vi "Base_eleve.vi"() -> ()   [LabVIEW 2018]
uses:
  <vilib>/Instr/_visa.llb/VISA Configure Serial Port (Instr).vi
panel:
  out "Temperature (Kelvin)":dbl
  out "Temperature (Fahrenheit)":dbl
  in  "Chemin":path
  in  "Extension du fichier":string(combo)
  in  "Nom du fichier":string
  in  "OK Button":bool
  in  "PAUSE":bool
  out "Array 3":dbl[](array[numeric])
  out "Array 2":dbl[](array[numeric])
  out "Array":dbl[](array[numeric])
  out "Humidity":dbl[](graph)
  out "Pressure":dbl[](graph)
  out "Temperature":dbl[](graph)
  out "Humidity":dbl
  out "Pressure":dbl
  out "Temperature (Celsuis)":dbl
  out "Chaîne":string
  in  "stop":bool
  in  "Nom de ressource VISA":refnum<visa-resource-name>
  # "1. Brancher la carte Arduino sur un port USB\n2. Choisir le port COM de la carte dans la liste déroulante \"Nom de ressource VISA\"\n3. Lancer le programme"
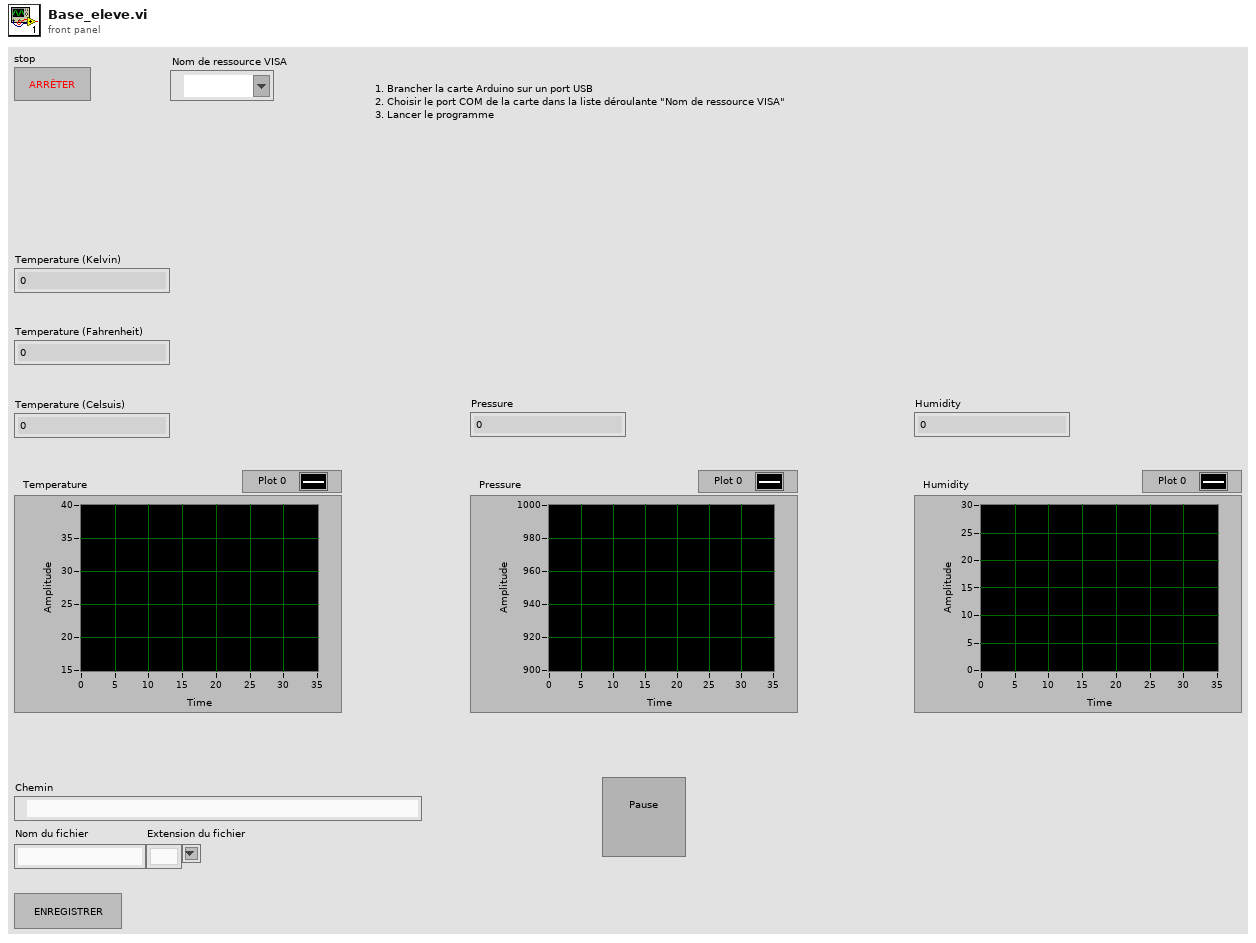
[diagram p1: front panel]
types:
  T1 = enum16{"open", "replace", "create", "open or create", "replace or create", "replace or create with confirmation"}
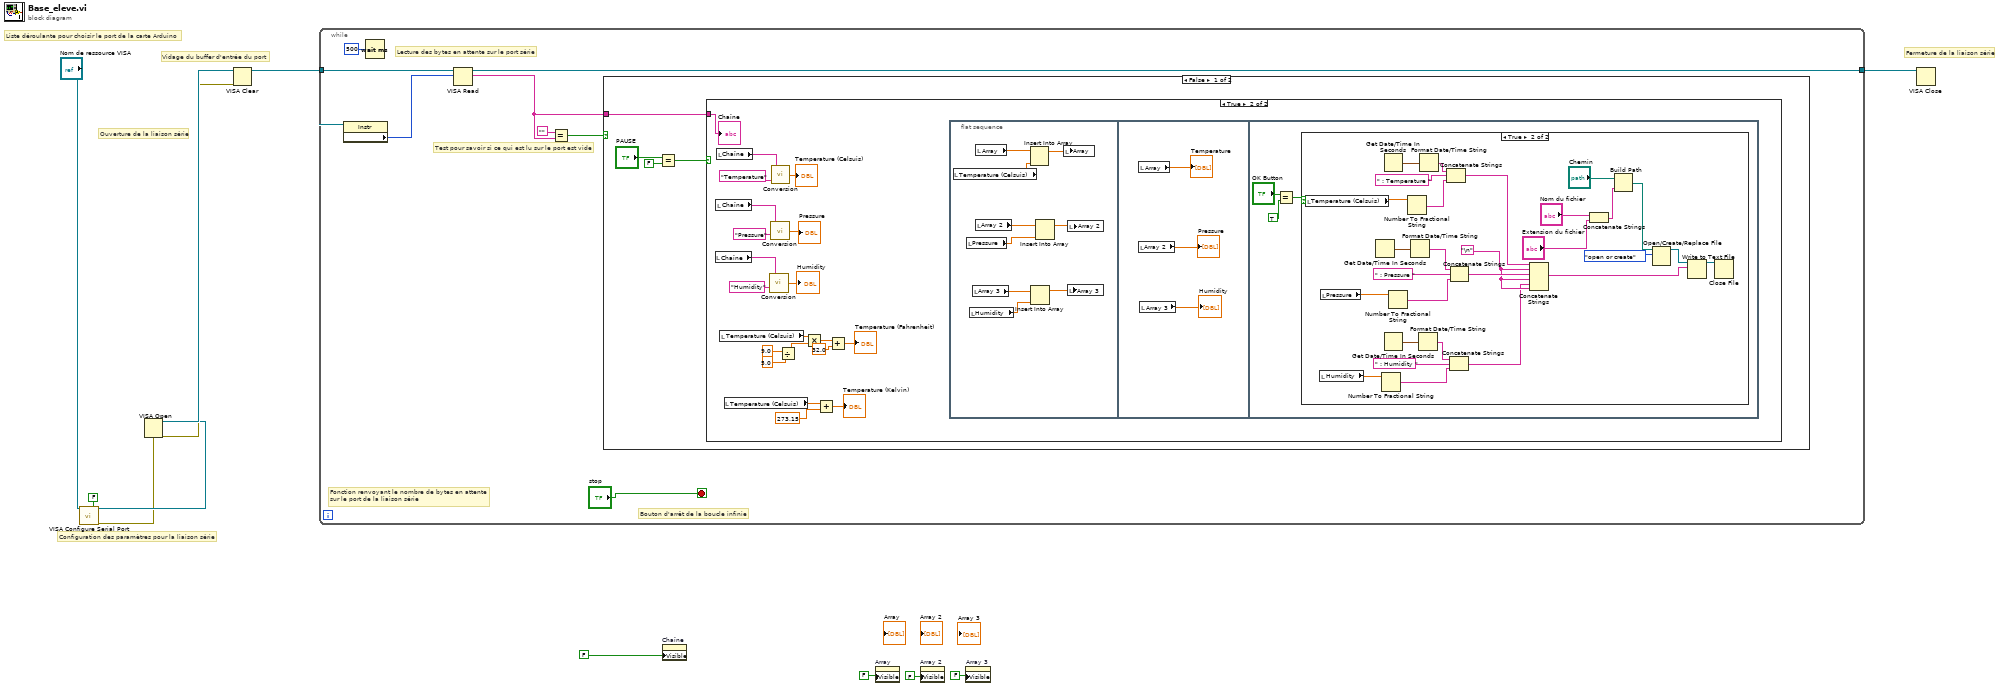
[diagram p0: block diagram]
diagram:
  # "Vidage du buffer d'entrée du port"
  # "Ouverture de la liaison série"
  # "Configuration des paramètres pour la liaison série"
  # "Liste déroulante pour choisir le port de la carte Arduino"
  # "Fermeture de la liaison série"
  n1 = call-poly "VISA Configure Serial Port"("VISA resource name"="Nom de ressource VISA", "Enable Termination\nChar (T)"=FALSE ("Enable Termination\nChar (T)")) -> ("VISA resource name out"=w9:refnum<visa-resource-name>, "error out"=w7:errorcluster)  [unwired: 12 in]
  n2 = VISA Open(error in (no error)=w7, VISA resource name=w9) -> (VISA resource name=w11:refnum<visa-resource-name>, error out=w6:errorcluster)  [unwired: 3 in]
  n3 = VISA Clear(VISA resource name=w11, error in (no error)=w6) -> (VISA resource name out=w10:refnum<visa-resource-name>)  [unwired: 1 out]
  n4 = while {
    tunnel: w10 -> [w20]
    tunnel: [w18] -> w5
    stop <- "stop" stop-if-true
    # "Lecture des bytes en attente sur le port série"
    # "Fonction renvoyant le nombre de bytes en attente\nsur le port de la liaison série"
    # "Test pour savoir si ce qui est lu sur le port est vide"
    # "Bouton d'arrêt de la boucle infinie"
    n5 = property class="Instr"(reference=w20) -> ("Serial Settings:Number of Bytes at Serial Port"=w19:u32)  [unwired: 1 in, 2 out]
    n6 = Wait (ms)(milliseconds to wait=u32 500 ("attente (ms)")) -> ()  [unwired: 1 out]
    n7 = VISA Read(VISA resource name=w20, byte count=w19) -> (VISA resource name out=w18:refnum<visa-resource-name>, read buffer=w15:string)  [unwired: 1 in, 2 out]
    n8 = Equal?(x="", y=w15) -> (x = y?=w13:bool)
    n9 = case shown="False" w13 {
      tunnel: w15 -> [w22 _]
      frame False {
        n10 = Equal?(x="PAUSE", y=FALSE) -> (x = y?=w21:bool)
        n11 = case shown="True" w21 {
          tunnel: w22 -> [_ w44]
          frame False {
          }
          frame True {
            n12 = local read "Chaîne"() -> (w39:string)
            n13 = local read "Chaîne"() -> (w40:string)
            n14 = local read "Chaîne"() -> (w43:string)
            n15 = local read "Temperature (Celsuis)"() -> (w32:dbl)
            n16 = local read "Temperature (Celsuis)"() -> (w27:dbl)
            n17 = call "Conversion.vi"("String 3"="Humidity", "String"=w39) -> ("Numeric"=→"Humidity":dbl)
            n18 = call "Conversion.vi"("String 3"="Pressure", "String"=w40) -> ("Numeric"=→"Pressure":dbl)
            n19 = call "Conversion.vi"("String 3"="Temperature", "String"=w43) -> ("Numeric"=→"Temperature (Celsuis)":dbl)
            n20 = Divide(x=9.0, y=5.0) -> (x/y=w31:dbl)
            n21 = Multiply(x=w32, y=w31) -> (x*y=w30:dbl)
            n22 = Add(x=w27, y=273.15) -> (x+y=→"Temperature (Kelvin)":dbl)
            n23 = Add(x=w30, y=32.0) -> (x+y=→"Temperature (Fahrenheit)":dbl)
            n24 = flat-sequence {
              frame #0 {
                n25 = local read "Temperature (Celsuis)"() -> (w46:dbl)
                n26 = local read "Pressure"() -> (w50:dbl)
                n27 = local read "Humidity"() -> (w53:dbl)
                n28 = local read "Array 3"() -> (w51:dbl[])
                n29 = local read "Array 2"() -> (w48:dbl[])
                n30 = local read "Array"() -> (w45:dbl[])
                n31 = Insert Into Array(array=w45, new element=w46) -> (w47:dbl[])  [unwired: 1 in]
                n32 = Insert Into Array(array=w51, new element=w53) -> (w52:dbl[])  [unwired: 1 in]
                n33 = Insert Into Array(array=w48, new element=w50) -> (w49:dbl[])  [unwired: 1 in]
                n34 = local write "Array"(w47) -> ()
                n35 = local write "Array 3"(w52) -> ()
                n36 = local write "Array 2"(w49) -> ()
              }
              frame #1 {
                n37 = local read "Array 2"() -> (→"Pressure":dbl[])
                n38 = local read "Array"() -> (→"Temperature":dbl[])
                n39 = local read "Array 3"() -> (→"Humidity":dbl[])
              }
              frame #2 {
                n40 = Equal?(x="OK Button", y=TRUE) -> (x = y?=w58:bool)
                n41 = case shown="True" w58 {
                  frame False {
                  }
                  frame True {
                    w76 = "\n"
                    n42 = local read "Temperature (Celsuis)"() -> (w71:dbl)
                    n43 = local read "Humidity"() -> (w67:dbl)
                    n44 = local read "Pressure"() -> (w69:dbl)
                    n45 = Get Date/Time In Seconds() -> (seconds since 1Jan1904=w86:timestamp)
                    n46 = Number To Fractional String(number=w67) -> (F-format string=w66:string)  [unwired: 3 in]
                    n47 = Get Date/Time In Seconds() -> (seconds since 1Jan1904=w87:timestamp)
                    n48 = Get Date/Time In Seconds() -> (seconds since 1Jan1904=w85:timestamp)
                    n49 = Number To Fractional String(number=w69) -> (F-format string=w68:string)  [unwired: 3 in]
                    n50 = Number To Fractional String(number=w71) -> (F-format string=w70:string)  [unwired: 3 in]
                    n51 = Format Date/Time String(seconds (now)=w86) -> (date/time string=w82:string)  [unwired: 2 in]
                    n52 = Format Date/Time String(seconds (now)=w85) -> (date/time string=w80:string)  [unwired: 2 in]
                    n53 = Format Date/Time String(seconds (now)=w87) -> (date/time string=w84:string)  [unwired: 2 in]
                    n54 = Concatenate Strings(w84, " : Temperature ", w70) -> (w78:string)
                    n55 = Concatenate Strings(w80, " : Humidity ", w66) -> (w75:string)
                    n56 = Concatenate Strings(w82, " : Pressure ", w68) -> (w77:string)
                    n57 = Concatenate Strings(w78, w76, w77, w76, w75, w76) -> (w62:string)
                    n58 = Concatenate Strings("Nom du fichier", "Extension du fichier") -> (w73:string)
                    n59 = Build Path(base path="Chemin", name or relative path=w73) -> (appended path=w64:path)
                    n60 = Open/Create/Replace File(file path (use dialog)=w64, operation (0:open)=T1."open or create") -> (refnum out=w63:refnum<file>)  [unwired: 4 in, 2 out]
                    n61 = Write to Text File(file (use dialog)=w63, text=w62) -> (refnum out=w60:refnum<file>)  [unwired: 2 in, 2 out]
                    n62 = Close File(refnum=w60) -> ()  [unwired: 1 in, 2 out]
                  }
                }
              }
            }
            "Chaîne" <- w44
          }
        }
      }
      frame True {
      }
    }
  }
  n63 = property on="Chaîne" class="Str"("Visible"=FALSE) -> ()  [unwired: 2 in, 2 out]
  n64 = property on="Array" class="Arr (strict)"("Visible"=FALSE) -> ()  [unwired: 2 in, 2 out]
  n65 = property on="Array 2" class="Arr (strict)"("Visible"=FALSE) -> ()  [unwired: 2 in, 2 out]
  n66 = property on="Array 3" class="Arr (strict)"("Visible"=FALSE) -> ()  [unwired: 2 in, 2 out]
  n67 = VISA Close(VISA resource name=w5) -> ()  [unwired: 1 in, 1 out]
